vi "BooleanToggle.vi"(11 "Input":bool) -> (3 "Output":bool)   [LabVIEW 2014]
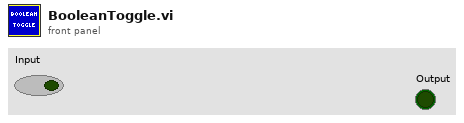
[diagram p1: front panel]
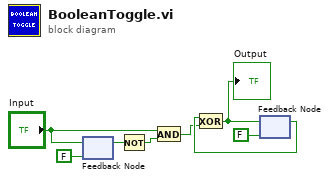
[diagram p0: block diagram]
diagram:
  n1 = feedback-in #1("Input") -> ()
  n2 = feedback #1(FALSE ("Input")) -> (w6:bool)
  n3 = Not(x=w6) -> (.not. x?=w5:bool)
  n4 = And(x="Input", y=w5) -> (x .and. y?=w2:bool)
  n5 = feedback #2(FALSE) -> (w3:bool)
  n6 = Exclusive Or(1:w2, 2:w3) -> (0:w1:bool)
  "Output" <- w1
  n7 = feedback-in #2(w1) -> ()
